vi "dvr_fgv_read.vi"(8 "error in (no error)":errorcluster) -> (0 "error out":errorcluster, 3 "Boolean":bool)   [LabVIEW 2020]
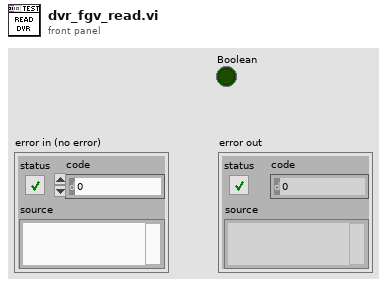
[diagram p1: front panel]
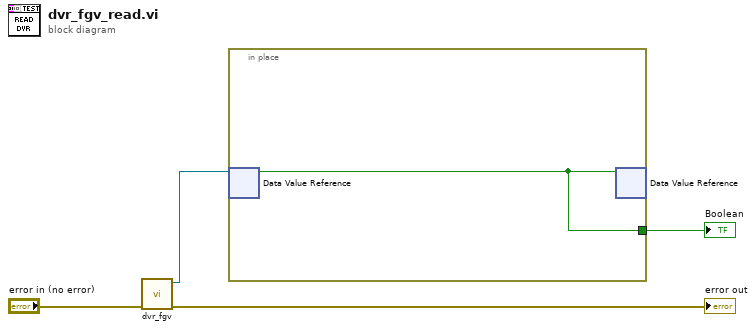
[diagram p0: block diagram]
diagram:
  n1 = call "dvr_fgv.vi"("error in (no error)"="error in (no error)") -> ("error out"=→"error out":errorcluster, "data value reference"=w2:refnum<data-value>)  [unwired: 9 in]
  n2 = in-place {
    in-place-border: [w5] -> w1
    n3 = in-place-dvr #1(w2) -> (w5:bool)  [unwired: 1 out]
    n4 = in-place-dvr #1(w5) -> ()  [unwired: 2 out]
  }
  "Boolean" <- w1
